vi "Begin.vi"(8 "error in (no error)":errorcluster, 11 "Vision in":refnum<class "Vision.lvclass">) -> (0 "error out":errorcluster, 3 "Vision out":refnum<class "Vision.lvclass">)   [LabVIEW 2018, in "Vision.lvlib" / "Vision.lvclass"]
uses:
  Vision.lvclass
  <vilib>/Rock Robotics/Network Tables/NT Write Number.vi
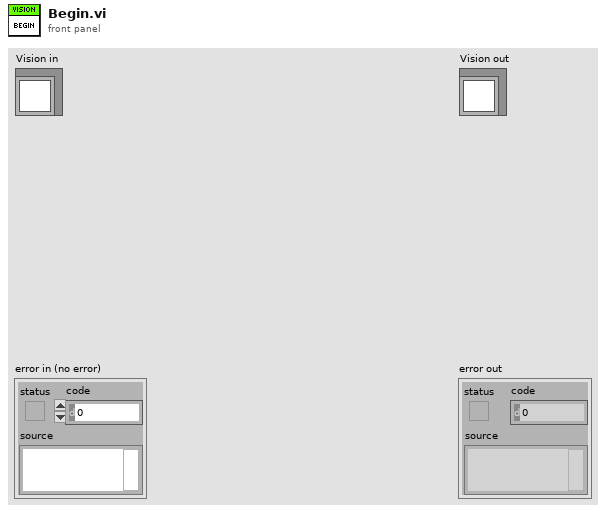
[diagram p1: front panel]
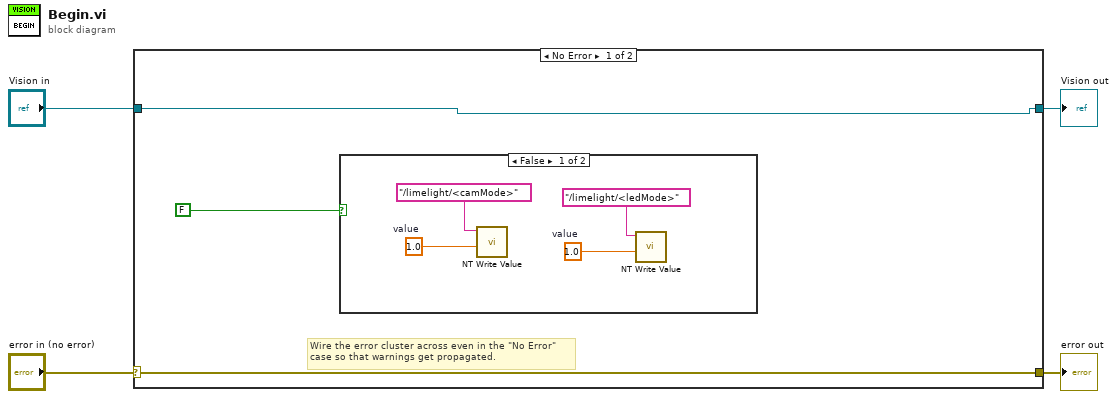
[diagram p0: block diagram]
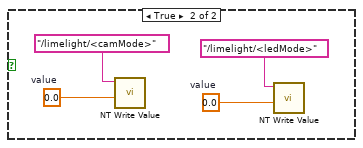
[diagram p2: hidden frame]
diagram:
  n1 = case shown="No Error" "error in (no error)" {
    selector: "error in (no error)" -> [w7 w17]
    tunnel: [w7 w17] -> w3
    tunnel: [w6 w16] -> w1
    tunnel: "Vision in" -> [w6 w16]
    frame No Error {
      # "Wire the error cluster across even in the \"No Error\"\ncase so that warnings get propagated."
      n2 = case shown="False" FALSE ("Vision Procesing Mode?") {
        frame False {
          w9 = 1.0  # value
          w11 = 1.0  # value
          n3 = call-poly <vilib>:"NT Write Value.vi"("Numeric"=w11, "Name"="/limelight/<camMode>") -> ()  [unwired: 9 in, 1 out]
          n4 = call-poly <vilib>:"NT Write Value.vi"("Numeric"=w9, "Name"="/limelight/<ledMode>") -> ()  [unwired: 9 in, 1 out]
        }
        frame True {
          w13 = 0.0  # value
          w15 = 0.0  # value
          n5 = call-poly <vilib>:"NT Write Value.vi"("Numeric"=w15, "Name"="/limelight/<camMode>") -> ()  [unwired: 9 in, 1 out]
          n6 = call-poly <vilib>:"NT Write Value.vi"("Numeric"=w13, "Name"="/limelight/<ledMode>") -> ()  [unwired: 9 in, 1 out]
        }
      }
    }
    frame Error {
    }
  }
  "error out" <- w3
  "Vision out" <- w1
